vi "Write Message.vi"(8 "error in (no error)":errorcluster, 9 "Message Contents":string, 10 "Message Type":string, 11 "CLI in":refnum<class "CLI.lvclass">) -> (0 "error out":errorcluster, 3 "CLI out":refnum<class "CLI.lvclass">)   [LabVIEW 2015, in "CLI.lvclass"]
uses:
  CLI.lvclass
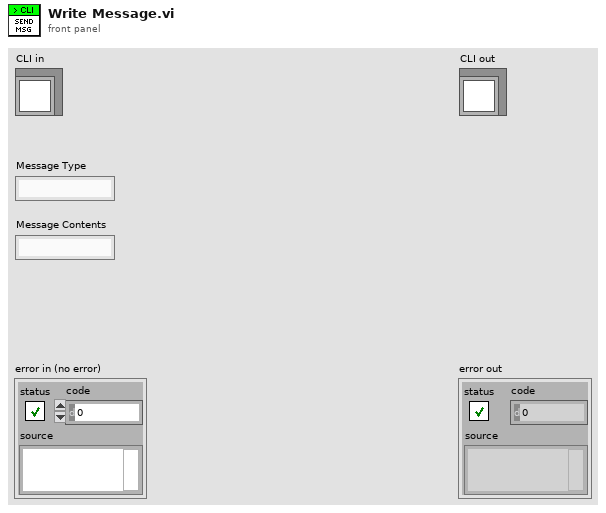
[diagram p1: front panel]
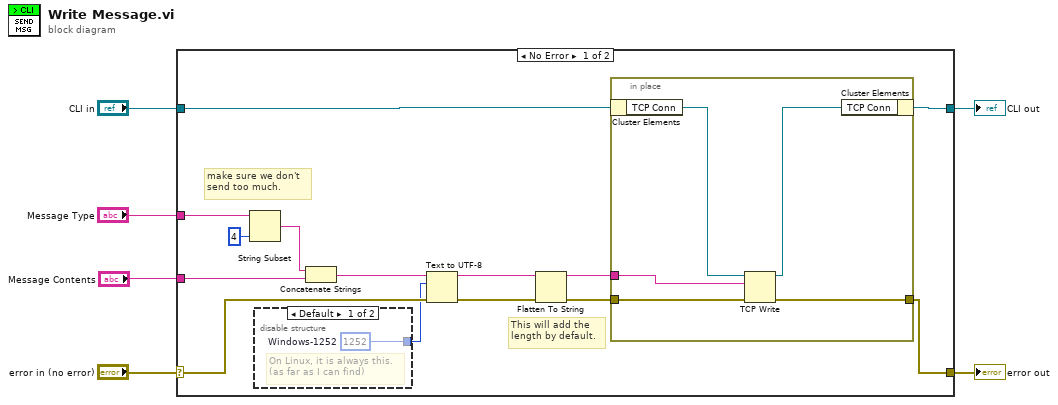
[diagram p0: block diagram]
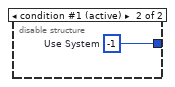
[diagram p2: hidden frame]
diagram:
  n1 = case shown="No Error" "error in (no error)" {
    selector: "error in (no error)" -> [w8 w29]
    tunnel: [w14 w29] -> w5
    tunnel: [w12 w28] -> w3
    tunnel: "CLI in" -> [w16 w28]
    tunnel: "Message Type" -> [w20 _]
    tunnel: "Message Contents" -> [w17 _]
    frame No Error {
      # "This will add the\nlength by default."
      # "make sure we don't\nsend too much."
      n2 = String Subset(string=w20, length (rest)=4 ("length (rest)")) -> (substring=w18:string)  [unwired: 1 in]
      n3 = disable-structure shown="Default" {
        disable-tunnel: [w21 w22] -> w7
        frame condition #0 {
          w21 = 1252  # Windows-1252
          # "On Linux, it is always this.\n(as far as I can find)"
        }
        frame condition #1 (active) {
          w22 = -1  # Use System
        }
      }
      n4 = Concatenate Strings(w18, w17) -> (w9:string)
      n5 = Text to UTF-8(8:w8, 10:w7, 11:w9) -> (0:w10:errorcluster, 3:w11:string)
      n6 = Flatten To String(anything=w11, error in (no error)=w10) -> (data string=w13:string, error out=w15:errorcluster)  [unwired: 2 in, 1 out]
      n7 = in-place {
        in-place-border: w15 -> [w26]
        in-place-border: [w25] -> w14
        in-place-border: w13 -> [w24]
        n8 = in-place-cluster #1(w16) -> ("TCP Conn"=w27:refnum<k5>)
        n9 = TCP Write(connection ID=w27, data in=w24, error in (no error)=w26) -> (connection ID out=w23:refnum<k5>, error out=w25:errorcluster)  [unwired: 1 in, 1 out]
        n10 = in-place-cluster #1("TCP Conn"=w23) -> (w12:refnum<class "CLI.lvclass">)
      }
    }
    frame Error {
    }
  }
  "error out" <- w5
  "CLI out" <- w3
